vi "f(x) quadratic model.vi"() -> ()   [LabVIEW 2009]
uses:
  polynomial equation.ctl
panel:
  out "Array 2":bool[](array[boolean])
  out "substitution results":T1[](array[typedef])
  out "eelimiation results":T1[](array[typedef])
  out "3 systems of eqations":T1[](array[typedef])
  in  "points":cluster{"x":dbl, "f(x)":dbl}[](array[cluster])
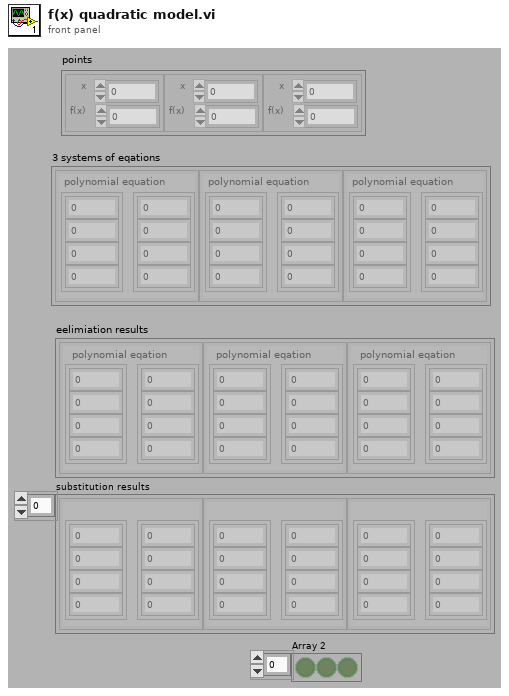
[diagram p1: front panel]
types:
  T1 = typedef "polynomial equation.ctl" = cluster{"i":dbl[], "ii":dbl[]}
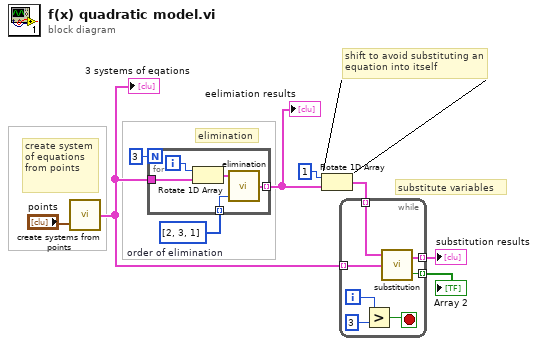
[diagram p0: block diagram]
diagram:
  w7 = i32[] [2, 3, 1]  # order of elimination
  # "substitute variables"
  # "shift to avoid substituting an equation into itself"
  # "elimination"
  # "create system  of equations from points"
  n1 = call "create systems from points.vi"("points"="points") -> ("systems of equations"=w3:T1[])  [unwired: 1 in]
  "3 systems of eqations" <- w3
  n2 = for {
    N: 3 -> [_]
    tunnel: w3 -> [w14]
    tunnel: [w12] -> w4 mode=indexing
    tunnel: w7 -> [w11] mode=indexing
    i -> [w10]
    n3 = Rotate 1D Array(1:w14, 2:w10) -> (0:w13:T1[])
    n4 = call "elimination.vi"("index to compare"=w11, "input equations"=w13) -> ("x-y"=w12:T1)  [unwired: 3 in]
  }
  "eelimiation results" <- w4
  n5 = Rotate 1D Array(1:w4, 2:1) -> (0:w5:T1[])
  n6 = while {
    tunnel: w5 -> [w16] mode=indexing
    tunnel: w3 -> [w15] mode=indexing
    tunnel: [w21] -> w2 mode=indexing
    tunnel: [w20] -> w1 mode=indexing
    i -> [w17]
    stop <- w19 stop-if-true
    n7 = Greater?(x=w17, y=3 ("x")) -> (0:w19:bool)
    n8 = call "substitution.vi"("polynomial equation 2"=w15, "polynomial equation 1"=w16) -> ("successful?"=w20:bool, "polynomial equation 1"=w21:T1)  [unwired: 2 in]
  }
  "substitution results" <- w2
  "Array 2" <- w1
